vi "XY Graph Get X Scales Grid Colors.vi"(8 "error in (no error)":errorcluster, 11 "XYGraph in":T1) -> (0 "error out":errorcluster, 1 "Was Tag Found?":bool, 2 "X Scale.Grid Colors":cluster{"Major Color":u32, "Minor Color":u32}[](array[cluster]), 3 "XYGraph out":T1)   [LabVIEW 2019, in "XY Graph Add-Ons.lvlib"]
uses:
  XY Graph Add-Ons.lvlib
  XY Graph Refnum.ctl
  XY Graph Property Tag List.ctl
  <vilib>/UserTags/UserTags.lvlib
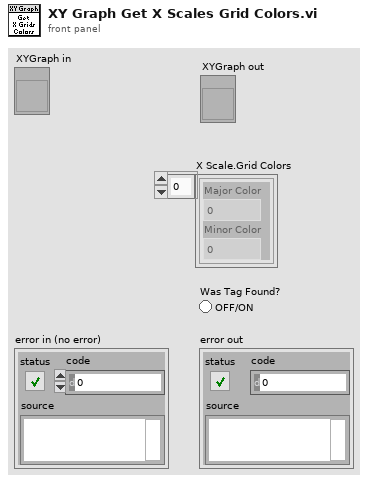
[diagram p1: front panel]
types:
  T1 = typedef "XY Graph Add-Ons.lvlib/XY Graph Refnum.ctl" = refnum<vi>
  T2 = typedef "XY Graph Add-Ons.lvlib/XY Graph Property Tag List.ctl" = enum16{"Max Legend Size", "Preserved Plots", "XScales.GridColors", "YScales.GridColors", "TipStrip String", "TipStrip Visible", "Tool Panels Visibility", "Plots Metadata"}
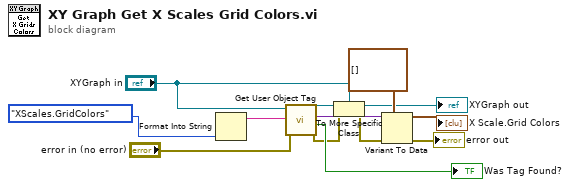
[diagram p0: block diagram]
diagram:
  n1 = Format Into String(XY_Graph_Property_Tag_List."XScales.GridColors" ("XY Graph Property Tag")) -> (resulting string=w12:string)  [unwired: 3 in, 1 out]
  n2 = call <vilib>:"Get User Object Tag.vi"("error in (no error)"="error in (no error)", "Tag Name"=w12, "Generic Refnum"="XYGraph in") -> ("error out"=w3:errorcluster, "Was Tag Found?"=→"Was Tag Found?":bool, "Value"=w9:variant, "dup Generic Refnum"=w6:refnum<vi>)  [unwired: 5 in]
  n3 = To More Specific Class(target class="XYGraph in", reference=w6, error in=w3) -> (specific class reference=→"XYGraph out":T1, error out=w2:errorcluster)
  n4 = Variant To Data(error in=w2, type=cluster{"Major Color":u32, "Minor Color":u32}[] [] ("X Scale.Grid Colors"), Variant=w9) -> (data=→"X Scale.Grid Colors":cluster{"Major Color":u32, "Minor Color":u32}[], error out=→"error out":errorcluster)
